vi "ASI_test221128.vi"() -> ()   [LabVIEW 2023]
uses:
  <vilib>/vision/Image Controls.llb/IMAQ Image.ctl
  user.lib/ASICamera2_no_err/ASICamera2_no_err.lvlib
panel:
  in  "live":bool
  out "New Image":T1
  out "Abort":bool
  in  "snap":bool
  in  "abort":bool
  in  "选项卡控件":enum32{"cool", "capture", "setting"}(tab)
  in  "cooler":bool
  in  "set point":i8
  in  "capture num":u16
  in  "imageType":u16(ring)
  in  "bin":u16(ring)
  out "temp and cool chart":cluster{dbl, "plValue out":i32}(graph)
  out "IsCoolerCam":u32
  out "exit":bool
  out "exposure progress":u8(slide) scale=0.0..100.0
  in  "clear ROI":bool
  in  "ROI":bool
  in  "OldCtrlVal[]":cluster{"value":dbl, "auto":bool}[](array[cluster]) {"value" min=-500.0 max=1000.0}
  in  "clusterOldCtrlVal":cluster{"value":dbl, "auto":bool} {"value" min=-500.0 max=1000.0}
  in  "cluster_controlCap":T2
  in  "controlCaps[]":T3(array[cluster])
  out "camera name":string
  in  "newCtrlVal[]":T4(array[cluster])
  in  "cluster":cluster{"name":string, "value":dbl, "auto":bool} {"value" min=-500.0 max=1000.0}
  out "Image":T1(plugin-control)
  out "CameraID":i32
  out "MaxWidth":i32
  out "MaxHeight":i32
  in  "Exit":bool
  in  "iCameraIndex":i32
  out "camera num":i32
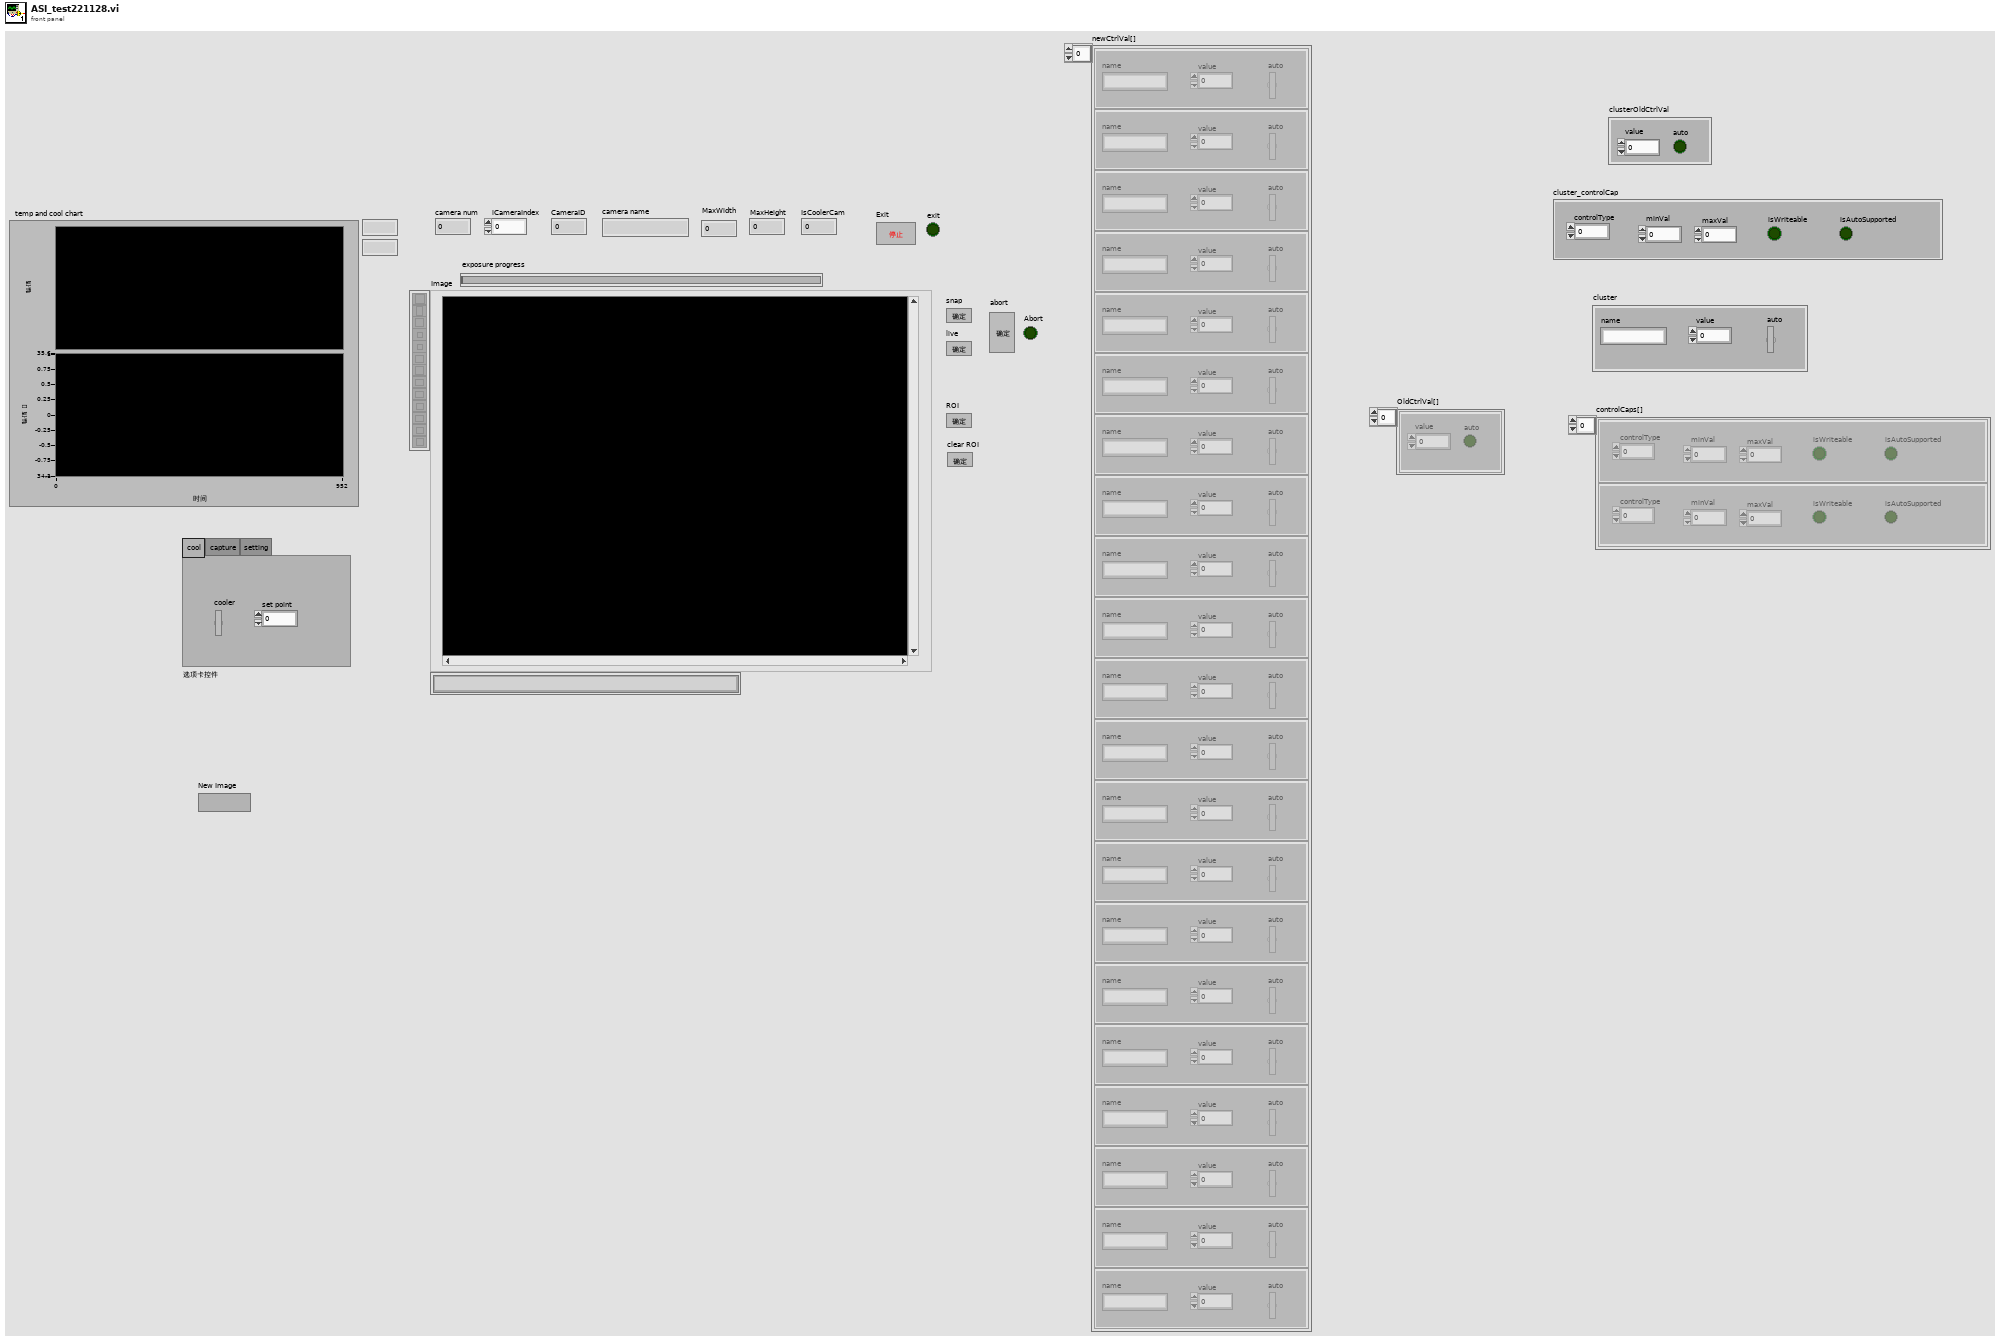
[diagram p1: front panel]
types:
  T1 = typedef "IMAQ Image.ctl" = refnum<image>
  T2 = cluster{"minVal":dbl, "maxVal":dbl, "isWriteable":bool, "isAutoSupported":bool, "controlType":dbl}
  T3 = cluster{"minVal":dbl, "maxVal":dbl, "isWriteable":bool, "isAutoSupported":bool, "controlType":dbl}[]
  T4 = cluster{"name":string, "value":dbl, "auto":bool}[]
  T5 = cluster{"Name[0]":i8, "Name[1]":i8, "Name[2]":i8, "Name[3]":i8, "Name[4]":i8, "Name[5]":i8, "Name[6]":i8, "Name[7]":i8, "Name[8]":i8, "Name[9]":i8, "Name[10]":i8, "Name[11]":i8, "Name[12]":i8, "Name[13]":i8, "Name[14]":i8, "Name[15]":i8, "Name[16]":i8, "Name[17]":i8, "Name[18]":i8, "Name[19]":i8, "Name[20]":i8, "Name[21]":i8, "Name[22]":i8, "Name[23]":i8, "Name[24]":i8, "Name[25]":i8, "Name[26]":i8, "Name[27]":i8, "Name[28]":i8, "Name[29]":i8, "Name[30]":i8, "Name[31]":i8, "Name[32]":i8, "Name[33]":i8, "Name[34]":i8, "Name[35]":i8, "Name[36]":i8, "Name[37]":i8, "Name[38]":i8, "Name[39]":i8, "Name[40]":i8, "Name[41]":i8, "Name[42]":i8, "Name[43]":i8, "Name[44]":i8, "Name[45]":i8, "Name[46]":i8, "Name[47]":i8, "Name[48]":i8, "Name[49]":i8, "Name[50]":i8, "Name[51]":i8, "Name[52]":i8, "Name[53]":i8, "Name[54]":i8, "Name[55]":i8, "Name[56]":i8, "Name[57]":i8, "Name[58]":i8, "Name[59]":i8, "Name[60]":i8, "Name[61]":i8, "Name[62]":i8, "Name[63]":i8, "CameraID":i32, "MaxHeight":i32, "MaxWidth":i32, "IsColorCam":u32, "BayerPattern":u32, "SupportedBins[0]":i32, "SupportedBins[1]":i32, "SupportedBins[2]":i32, "SupportedBins[3]":i32, "SupportedBins[4]":i32, "SupportedBins[5]":i32, "SupportedBins[6]":i32, "SupportedBins[7]":i32, "SupportedBins[8]":i32, "SupportedBins[9]":i32, "SupportedBins[10]":i32, "SupportedBins[11]":i32, "SupportedBins[12]":i32, "SupportedBins[13]":i32, "SupportedBins[14]":i32, "SupportedBins[15]":i32, "SupportedVideoFormat[0]":u32, "SupportedVideoFormat[1]":u32, "SupportedVideoFormat[2]":u32, "SupportedVideoFormat[3]":u32, "SupportedVideoFormat[4]":u32, "SupportedVideoFormat[5]":u32, "SupportedVideoFormat[6]":u32, "SupportedVideoFormat[7]":u32, "@dummy control@":i8, "@dummy control@":i8, "@dummy control@":i8, "@dummy control@":i8, "PixelSize":dbl, "MechanicalShutter":u32, "ST4Port":u32, "IsCoolerCam":u32, "IsUSB3Host":u32, "IsUSB3Camera":u32, "ElecPerADU":sgl, "Unused[0]":i8, "Unused[1]":i8, "Unused[2]":i8, "Unused[3]":i8, "Unused[4]":i8, "Unused[5]":i8, "Unused[6]":i8, "Unused[7]":i8, "Unused[8]":i8, "Unused[9]":i8, "Unused[10]":i8, "Unused[11]":i8, "Unused[12]":i8, "Unused[13]":i8, "Unused[14]":i8, "Unused[15]":i8, "Unused[16]":i8, "Unused[17]":i8, "Unused[18]":i8, "Unused[19]":i8, "Unused[20]":i8, "Unused[21]":i8, "Unused[22]":i8, "Unused[23]":i8}
  T6 = typedef "Image Type" = u32
  T7 = cluster{"Name[0]":i8, "Name[1]":i8, "Name[2]":i8, "Name[3]":i8, "Name[4]":i8, "Name[5]":i8, "Name[6]":i8, "Name[7]":i8, "Name[8]":i8, "Name[9]":i8, "Name[10]":i8, "Name[11]":i8, "Name[12]":i8, "Name[13]":i8, "Name[14]":i8, "Name[15]":i8, "Name[16]":i8, "Name[17]":i8, "Name[18]":i8, "Name[19]":i8, "Name[20]":i8, "Name[21]":i8, "Name[22]":i8, "Name[23]":i8, "Name[24]":i8, "Name[25]":i8, "Name[26]":i8, "Name[27]":i8, "Name[28]":i8, "Name[29]":i8, "Name[30]":i8, "Name[31]":i8, "Name[32]":i8, "Name[33]":i8, "Name[34]":i8, "Name[35]":i8, "Name[36]":i8, "Name[37]":i8, "Name[38]":i8, "Name[39]":i8, "Name[40]":i8, "Name[41]":i8, "Name[42]":i8, "Name[43]":i8, "Name[44]":i8, "Name[45]":i8, "Name[46]":i8, "Name[47]":i8, "Name[48]":i8, "Name[49]":i8, "Name[50]":i8, "Name[51]":i8, "Name[52]":i8, "Name[53]":i8, "Name[54]":i8, "Name[55]":i8, "Name[56]":i8, "Name[57]":i8, "Name[58]":i8, "Name[59]":i8, "Name[60]":i8, "Name[61]":i8, "Name[62]":i8, "Name[63]":i8, "Description[0]":i8, "Description[1]":i8, "Description[2]":i8, "Description[3]":i8, "Description[4]":i8, "Description[5]":i8, "Description[6]":i8, "Description[7]":i8, "Description[8]":i8, "Description[9]":i8, "Description[10]":i8, "Description[11]":i8, "Description[12]":i8, "Description[13]":i8, "Description[14]":i8, "Description[15]":i8, "Description[16]":i8, "Description[17]":i8, "Description[18]":i8, "Description[19]":i8, "Description[20]":i8, "Description[21]":i8, "Description[22]":i8, "Description[23]":i8, "Description[24]":i8, "Description[25]":i8, "Description[26]":i8, "Description[27]":i8, "Description[28]":i8, "Description[29]":i8, "Description[30]":i8, "Description[31]":i8, "Description[32]":i8, "Description[33]":i8, "Description[34]":i8, "Description[35]":i8, "Description[36]":i8, "Description[37]":i8, "Description[38]":i8, "Description[39]":i8, "Description[40]":i8, "Description[41]":i8, "Description[42]":i8, "Description[43]":i8, "Description[44]":i8, "Description[45]":i8, "Description[46]":i8, "Description[47]":i8, "Description[48]":i8, "Description[49]":i8, "Description[50]":i8, "Description[51]":i8, "Description[52]":i8, "Description[53]":i8, "Description[54]":i8, "Description[55]":i8, "Description[56]":i8, "Description[57]":i8, "Description[58]":i8, "Description[59]":i8, "Description[60]":i8, "Description[61]":i8, "Description[62]":i8, "Description[63]":i8, "Description[64]":i8, "Description[65]":i8, "Description[66]":i8, "Description[67]":i8, "Description[68]":i8, "Description[69]":i8, "Description[70]":i8, "Description[71]":i8, "Description[72]":i8, "Description[73]":i8, "Description[74]":i8, "Description[75]":i8, "Description[76]":i8, "Description[77]":i8, "Description[78]":i8, "Description[79]":i8, "Description[80]":i8, "Description[81]":i8, "Description[82]":i8, "Description[83]":i8, "Description[84]":i8, "Description[85]":i8, "Description[86]":i8, "Description[87]":i8, "Description[88]":i8, "Description[89]":i8, "Description[90]":i8, "Description[91]":i8, "Description[92]":i8, "Description[93]":i8, "Description[94]":i8, "Description[95]":i8, "Description[96]":i8, "Description[97]":i8, "Description[98]":i8, "Description[99]":i8, "Description[100]":i8, "Description[101]":i8, "Description[102]":i8, "Description[103]":i8, "Description[104]":i8, "Description[105]":i8, "Description[106]":i8, "Description[107]":i8, "Description[108]":i8, "Description[109]":i8, "Description[110]":i8, "Description[111]":i8, "Description[112]":i8, "Description[113]":i8, "Description[114]":i8, "Description[115]":i8, "Description[116]":i8, "Description[117]":i8, "Description[118]":i8, "Description[119]":i8, "Description[120]":i8, "Description[121]":i8, "Description[122]":i8, "Description[123]":i8, "Description[124]":i8, "Description[125]":i8, "Description[126]":i8, "Description[127]":i8, "MaxValue":i32, "MinValue":i32, "DefaultValue":i32, "IsAutoSupported":u32, "IsWritable":u32, "ControlType":u32, "Unused[0]":i8, "Unused[1]":i8, "Unused[2]":i8, "Unused[3]":i8, "Unused[4]":i8, "Unused[5]":i8, "Unused[6]":i8, "Unused[7]":i8, "Unused[8]":i8, "Unused[9]":i8, "Unused[10]":i8, "Unused[11]":i8, "Unused[12]":i8, "Unused[13]":i8, "Unused[14]":i8, "Unused[15]":i8, "Unused[16]":i8, "Unused[17]":i8, "Unused[18]":i8, "Unused[19]":i8, "Unused[20]":i8, "Unused[21]":i8, "Unused[22]":i8, "Unused[23]":i8, "Unused[24]":i8, "Unused[25]":i8, "Unused[26]":i8, "Unused[27]":i8, "Unused[28]":i8, "Unused[29]":i8, "Unused[30]":i8, "Unused[31]":i8}
  T8 = cluster{"Global Rectangle":i32[], "Contours":cluster{"Contour Type":u32, "ROI Type":u32, "Points":i32[]}[]}
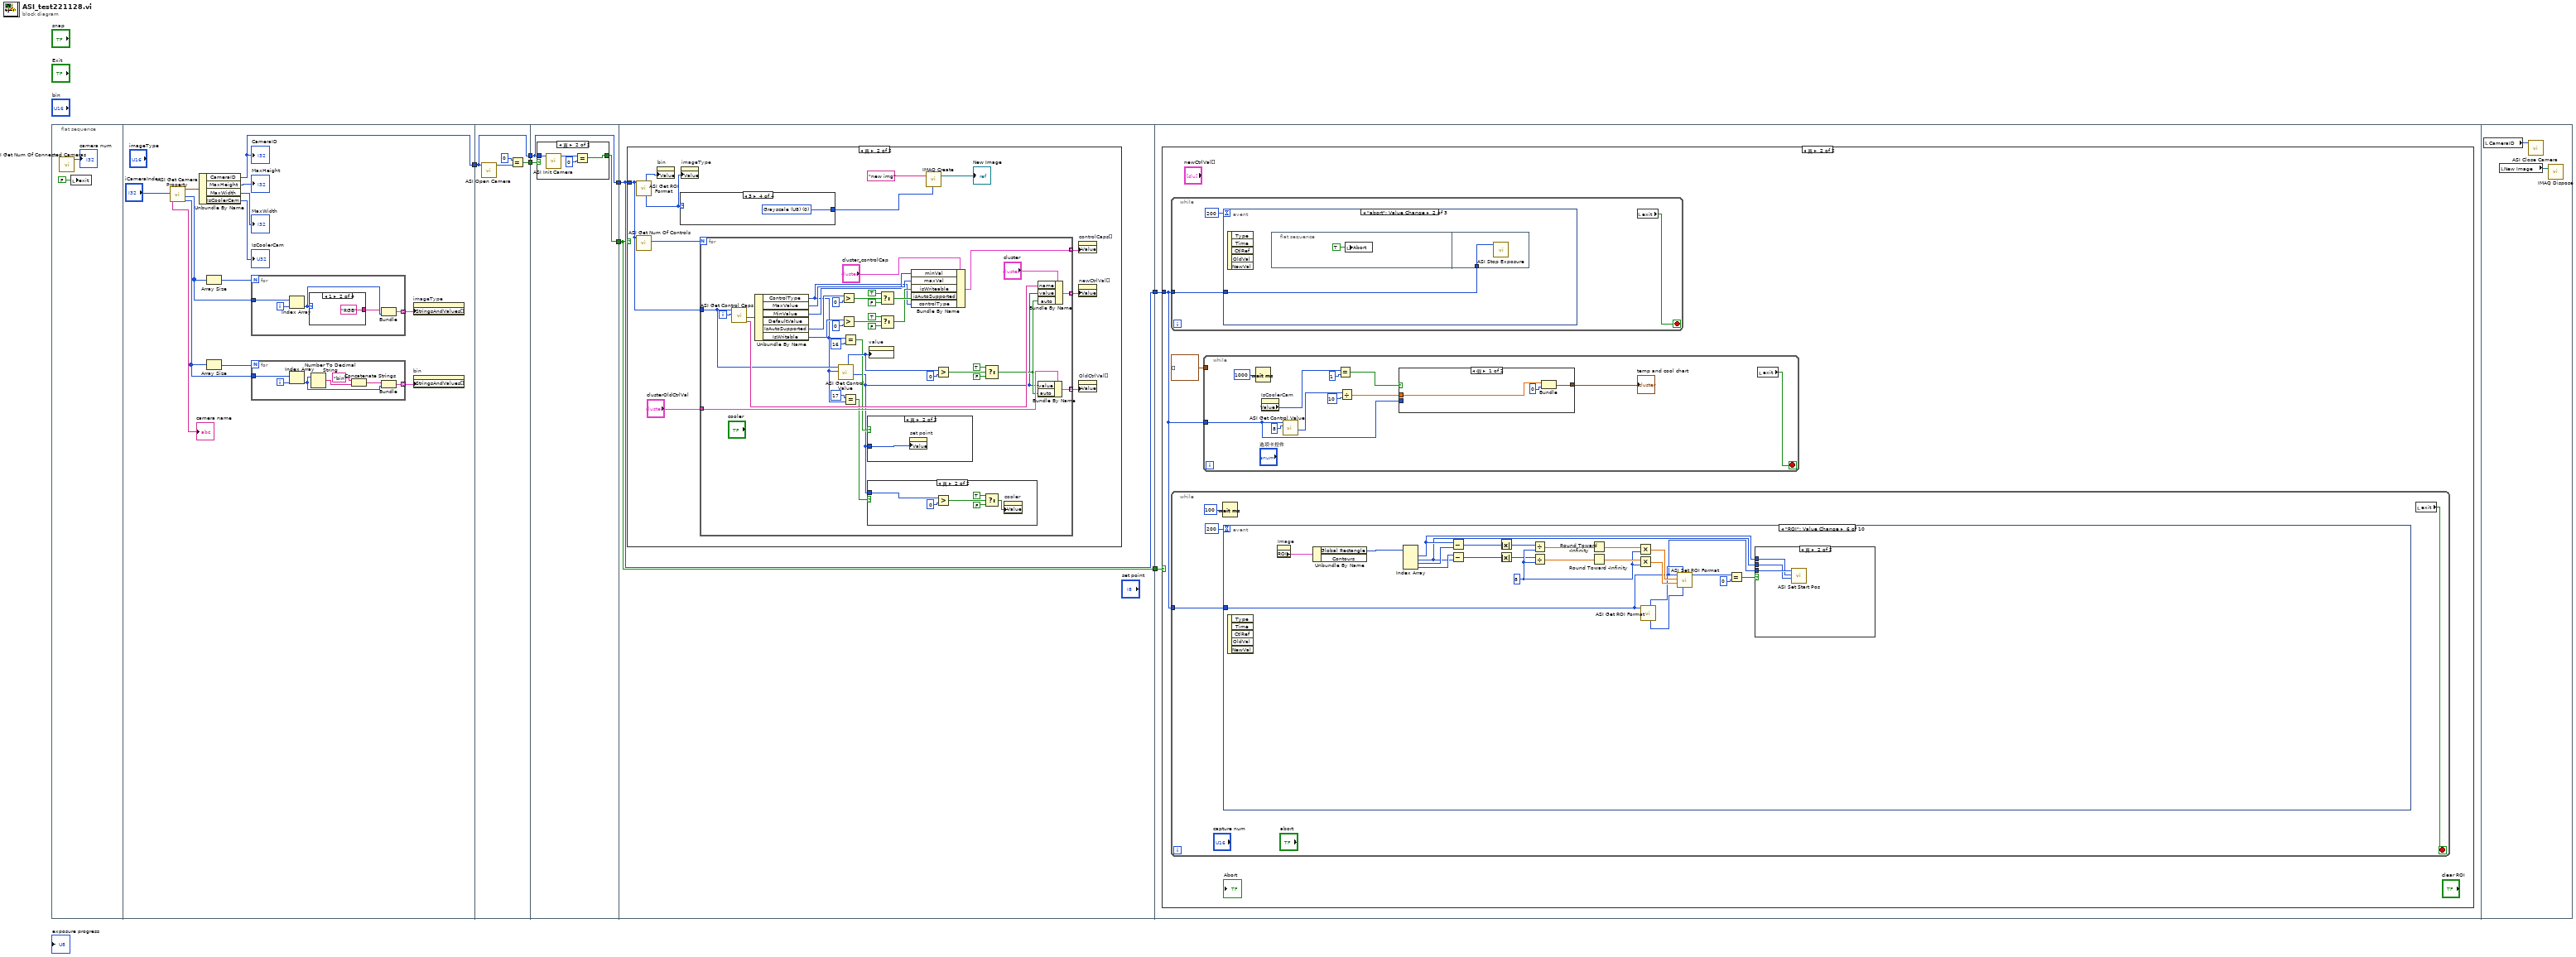
[diagram p0: block diagram]
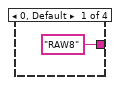
[diagram p2: hidden frame]
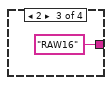
[diagram p3: hidden frame]
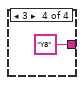
[diagram p4: hidden frame]
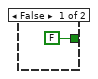
[diagram p5: hidden frame]
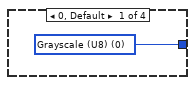
[diagram p7: hidden frame]
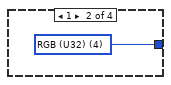
[diagram p8: hidden frame]
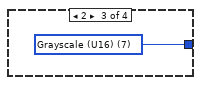
[diagram p9: hidden frame]
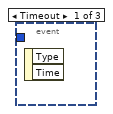
[diagram p13: hidden frame]
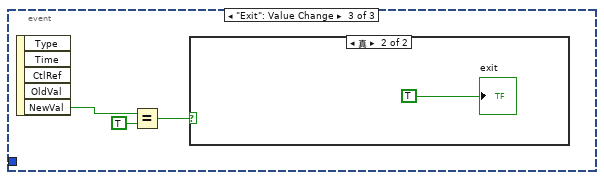
[diagram p14: hidden frame]
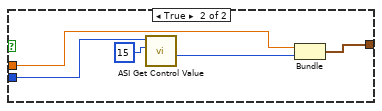
[diagram p16: hidden frame]
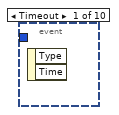
[diagram p17: hidden frame]
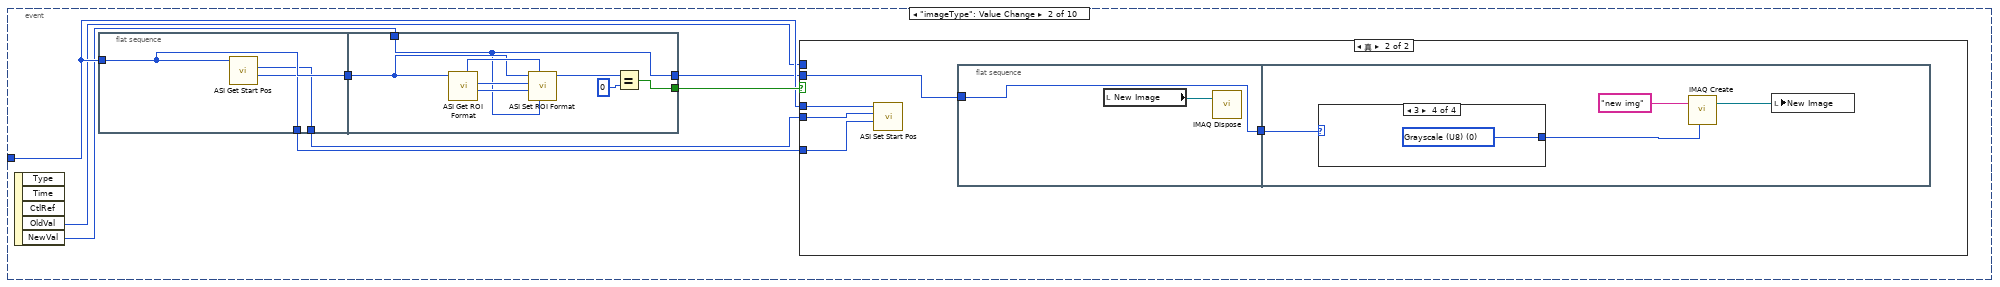
[diagram p18: hidden frame]
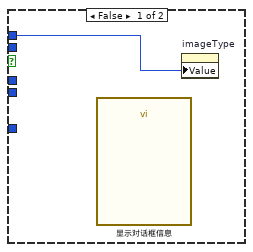
[diagram p19: hidden frame]
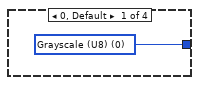
[diagram p20: hidden frame]
diagram:
  n1 = flat-sequence "平铺式顺序结构" {
    tunnel: [w20] -> w7
    tunnel: w7 -> [w42]
    tunnel: [w42] -> w6
    tunnel: [w39] -> w2
    tunnel: w6 -> [w45]
    tunnel: [w45] -> w5
    tunnel: w2 -> [w44]
    tunnel: [w43] -> w1
    tunnel: w5 -> [w52]
    tunnel: [w52] -> w4
    tunnel: [w51] -> w3
    tunnel: w1 -> [w51]
    tunnel: w4 -> [w112]
    tunnel: w3 -> [w111]
    frame #0 {
      n2 = call "ASI Get Num Of Connected Cameras.vi"() -> ("function return"=→"camera num":i32)  [unwired: 10 in, 1 out]
      n3 = local write "exit"(FALSE ("exit")) -> ()
    }
    frame #1 {
      n4 = call "ASI Get Camera Property.vi"("iCameraIndex"="iCameraIndex") -> ("supportedBin"=w15:i8[], "supportedImgType"=w16:i8[], "pASICameraInfo out"=w21:T5, "cameraName"=→"camera name":string)  [unwired: 6 in, 1 out]
      n5 = Unbundle By Name(w21) -> ("CameraID"=w20:i32, "MaxHeight"=→"MaxHeight":i32, "MaxWidth"=→"MaxWidth":i32, "IsCoolerCam"=→"IsCoolerCam":u32)
      "CameraID" <- w20
      n6 = Array Size(array=w16) -> (size(s)=w17:i32)
      n7 = Array Size(array=w15) -> (size(s)=w14:i32)
      n8 = for {
        N: w17 -> [_]
        tunnel: w16 -> [w33]
        tunnel: [w30] -> w11 mode=indexing
        i -> [w34]
        n9 = Index Array(array=w33, index=w34) -> (element=w32:i8)
        n10 = case shown="1" w32 {
          tunnel: ["RAW8" "RGB" "RAW16" "Y8"] -> w31
          frame 0, Default {
          }
          frame 1 {
          }
          frame 2 {
          }
          frame 3 {
          }
        }
        n11 = Bundle(w31, "SupportedVideoFormat[6]"=w32) -> (w30:cluster{string, "SupportedVideoFormat[6]":i8})  [unwired: 1 in]
      }
      n12 = for {
        N: w14 -> [_]
        tunnel: w15 -> [w28]
        tunnel: [w23] -> w13 mode=indexing
        i -> [w29]
        n13 = Index Array(array=w28, index=w29) -> (element=w27:i8)
        n14 = Number To Decimal String(number=w27) -> (decimal integer string=w25:string)  [unwired: 1 in]
        n15 = Concatenate Strings("bin" ("字符串"), w25) -> (w24:string)
        n16 = Bundle(w24, "元素"=w27) -> (w23:cluster{string, "元素":i8})  [unwired: 1 in]
      }
      n17 = property on="imageType" class="Ring (strict)"("StringsAndValues[]"=w11) -> ()  [unwired: 2 in, 2 out]
      n18 = property on="bin" class="Ring (strict)"("StringsAndValues[]"=w13) -> ()  [unwired: 2 in, 2 out]
    }
    frame #2 {
      n19 = call "ASI Open Camera.vi"("iCameraID"=w42) -> ("function return"=w41:i32)  [unwired: 10 in]
      n20 = Equal?(x=0, y=w41) -> (x = y?=w39:bool)
    }
    frame #3 {
      n21 = case shown="真" w44 {
        tunnel: w45 -> [_ w50]
        tunnel: [FALSE w47] -> w43
        frame False {
        }
        frame True {
          n22 = call "ASI Init Camera.vi"("iCameraID"=w50) -> ("function return"=w48:i32)  [unwired: 10 in]
          n23 = Equal?(x=w48, y=0 ("x")) -> (x = y?=w47:bool)
        }
      }
    }
    frame #4 {
      n24 = case shown="真" w51 {
        tunnel: w52 -> [_ w62]
        frame False {
        }
        frame True {
          n25 = call "ASI Get ROI Format.vi"("iCameraID"=w62) -> ("pImg_type out"=w54:i32, "piBin out"=w61:i32)  [unwired: 6 in, 3 out]
          n26 = call "ASI Get Num Of Controls.vi"("iCameraID"=w62) -> ("piNumberOfControls out"=w63:i32)  [unwired: 9 in, 1 out]
          n27 = property on="bin" class="Ring (strict)"("Value"=w61) -> ()  [unwired: 2 in, 2 out]
          n28 = case shown="3" w54 {
            tunnel: [w64 w65 w66 w67] -> w56
            frame 0, Default {
              w64 = T6 0 items=["Grayscale (U8)", "Grayscale (I16)", "Grayscale (SGL)", "Complex (CSG)", "RGB (U32)", "HSL (U32)", "RGB (U64)", "Grayscale (U16)"] ("Image Type")
            }
            frame 1 {
              w65 = T6 4 items=["Grayscale (U8)", "Grayscale (I16)", "Grayscale (SGL)", "Complex (CSG)", "RGB (U32)", "HSL (U32)", "RGB (U64)", "Grayscale (U16)"] ("Image Type")
            }
            frame 2 {
              w66 = T6 7 items=["Grayscale (U8)", "Grayscale (I16)", "Grayscale (SGL)", "Complex (CSG)", "RGB (U32)", "HSL (U32)", "RGB (U64)", "Grayscale (U16)"] ("Image Type")
            }
            frame 3 {
              w67 = T6 0 items=["Grayscale (U8)", "Grayscale (I16)", "Grayscale (SGL)", "Complex (CSG)", "RGB (U32)", "HSL (U32)", "RGB (U64)", "Grayscale (U16)"] ("Image Type")
            }
          }
          n29 = property on="imageType" class="Ring (strict)"("Value"=w54) -> ()  [unwired: 2 in, 2 out]
          n30 = for {
            N: w63 -> [_]
            tunnel: w62 -> [w100]
            tunnel: [w75] -> w60 mode=indexing
            tunnel: [w76] -> w59 mode=indexing
            tunnel: "clusterOldCtrlVal" -> [w79]
            tunnel: [w74] -> w57 mode=indexing
            i -> [w78]
            n31 = call "ASI Get Control Caps.vi"("iControlIndex"=w78, "iCameraID"=w100) -> ("name"=w101:string, "pControlCaps out"=w103:T7)  [unwired: 7 in, 1 out]
            n32 = Unbundle By Name(w103) -> ("ControlType"=w71:u32, "MaxValue"=w93:i32, "MinValue"=w92:i32, "IsAutoSupported"=w89:u32, "IsWritable"=w82:u32)  [unwired: 1 out]
            n33 = call "ASI Get Control Value.vi"("ControlType"=w71, "iCameraID"=w100) -> ("plValue out"=w68:i32, "pbAuto out"=w95:i32)  [unwired: 7 in, 1 out]
            n34 = Greater?(x=w89, y=u32 0) -> (0:w87:bool)
            n35 = Greater?(x=w82, y=u32 0) -> (0:w81:bool)
            n36 = Equal?(x=w71, y=u32 16) -> (x = y?=w69:bool)
            n37 = Equal?(x=u32 17, y=w71) -> (x = y?=w72:bool)
            n38 = case shown="真" w69 {
              tunnel: w68 -> [_ w104]
              frame False {
              }
              frame True {
                n39 = property on="set point" class="DigNum (strict)"("Value"=w104) -> ()  [unwired: 2 in, 2 out]
              }
            }
            n40 = case shown="真" w72 {
              tunnel: w68 -> [_ w106]
              frame False {
              }
              frame True {
                n41 = Greater?(x=w106, y=0) -> (0:w108:bool)
                n42 = Select(t=TRUE, s=w108, f=FALSE) -> (s? t:f=w105:bool)
                n43 = property on="cooler" class="Bool (strict)"("Value"=w105) -> ()  [unwired: 2 in, 2 out]
              }
            }
            n44 = property on="value" class="DigNum (strict)"("DisabledEnum"=w95) -> ()  [unwired: 2 in, 2 out]
            n45 = Select(t=TRUE, s=w87, f=FALSE) -> (s? t:f=w86:bool)
            n46 = Select(t=TRUE, s=w81, f=FALSE) -> (s? t:f=w80:bool)
            n47 = Bundle By Name(cluster="cluster_controlCap", "minVal"=w92, "maxVal"=w93, "isWriteable"=w80, "isAutoSupported"=w86, "controlType"=w71) -> (w76:T2)
            n48 = Greater?(x=w95, y=0) -> (0:w99:bool)
            n49 = Select(t=TRUE, s=w99, f=FALSE) -> (s? t:f=w77:bool)
            n50 = Bundle By Name(cluster="cluster", "name"=w101, "value"=w68, "auto"=w77) -> (w75:cluster{"name":string, "value":dbl, "auto":bool})
            n51 = Bundle By Name(cluster=w79, "value"=w68, "auto"=w77) -> (w74:cluster{"value":dbl, "auto":bool})
          }
          n52 = call "IMAQ Create"("Image Name"="new img", "Image Type"=w56) -> ("New Image"=→"New Image":T1)  [unwired: 3 in, 1 out]
          n53 = property on="controlCaps[]" class="Arr (strict)"("Value"=w59) -> ()  [unwired: 2 in, 2 out]
          n54 = property on="newCtrlVal[]" class="Arr (strict)"("Value"=w60) -> ()  [unwired: 2 in, 2 out]
          n55 = property on="OldCtrlVal[]" class="Arr (strict)"("Value"=w57) -> ()  [unwired: 2 in, 2 out]
        }
      }
    }
    frame #5 {
      n56 = case shown="真" w111 {
        tunnel: w112 -> [_ w114]
        frame False {
        }
        frame True {
          n57 = while {
            tunnel: w114 -> [w117]
            stop <- w115 stop-if-true
            n58 = event shown="[1] \"abort\": Value Change" {
              selector: _ -> [_ _ _]
              dyn-events: _ -> [_ _ _]
              timeout: 200 -> [_ _ _]
              tunnel: w117 -> [_ w118 _]
              event Timeout {
                n59 = event-data() -> ()  [unwired: 1 in, 2 out]
              }
              event "abort": Value Change {
                n60 = event-data() -> ()  [unwired: 1 in, 5 out]
                n61 = flat-sequence {
                  tunnel: w118 -> [w120]
                  frame #0 {
                    n62 = local write "Abort"(TRUE ("exit")) -> ()
                  }
                  frame #1 {
                    n63 = call "ASI Stop Exposure.vi"("iCameraID"=w120) -> ()  [unwired: 10 in, 1 out]
                  }
                }
              }
              event "Exit": Value Change {
                n64 = event-data() -> ("NewVal"=w123:bool)  [unwired: 1 in, 4 out]
                n65 = Equal?(x=w123, y=TRUE) -> (x = y?=w121:bool)
                n66 = case shown="真" w121 {
                  frame False {
                  }
                  frame True {
                    "exit" <- TRUE ("exit")
                  }
                }
              }
            }
            n67 = local read "exit"() -> (w115:bool)
          }
          n68 = while {
            tunnel: w114 -> [w146]
            stop <- w144 stop-if-true
            n69 = Wait (ms)(milliseconds to wait=u32 100 ("等待时间（毫秒）")) -> ()  [unwired: 1 out]
            n70 = event shown="[5] \"ROI\": Value Change" {
              selector: _ -> [_ _ _ _ _ _ _ _ _ _]
              dyn-events: _ -> [_ _ _ _ _ _ _ _ _ _]
              timeout: 200 -> [_ _ _ _ _ _ _ _ _ _]
              tunnel: w146 -> [_ w154 w186 w218 w272 w314 w347 w358 w367 w373]
              event Timeout {
                n71 = event-data() -> ()  [unwired: 1 in, 2 out]
              }
              event "imageType": Value Change {
                n72 = event-data() -> ("OldVal"=w149:u16, "NewVal"=w150:u16)  [unwired: 1 in, 3 out]
                n73 = flat-sequence {
                  tunnel: w154 -> [w158]
                  tunnel: [w158] -> w153
                  tunnel: [w157] -> w152
                  tunnel: [w156] -> w151
                  tunnel: [w162] -> w155
                  tunnel: w153 -> [w160]
                  tunnel: w150 -> [w159]
                  tunnel: [w159] -> w148
                  frame #0 {
                    n74 = call "ASI Get Start Pos.vi"("iCameraID"=w158) -> ("piStartY out"=w156:i32, "piStartX out"=w157:i32)  [unwired: 8 in, 1 out]
                  }
                  frame #1 {
                    n75 = call "ASI Get ROI Format.vi"("iCameraID"=w160) -> ("piHeight out"=w165:i32, "piWidth out"=w166:i32, "piBin out"=w164:i32)  [unwired: 6 in, 2 out]
                    n76 = call "ASI Set ROI Format.vi"("Img_type"=w159, "iBin"=w164, "iHeight"=w165, "iWidth"=w166, "iCameraID"=w160) -> ("function return"=w161:i32)  [unwired: 6 in]
                    n77 = Equal?(x=w161, y=u8 0) -> (x = y?=w162:bool)
                  }
                }
                n78 = case shown="真" w155 {
                  tunnel: w154 -> [_ w172]
                  tunnel: w152 -> [_ w171]
                  tunnel: w151 -> [_ w170]
                  tunnel: w149 -> [w167 _]
                  tunnel: w148 -> [_ w169]
                  frame False {
                    n79 = call "显示对话框信息"() -> ()  [unwired: 10 in, 2 out]
                    n80 = property on="imageType" class="Ring (strict)"("Value"=w167) -> ()  [unwired: 2 in, 2 out]
                  }
                  frame True {
                    n81 = call "ASI Set Start Pos.vi"("iStartY"=w170, "iStartX"=w171, "iCameraID"=w172) -> ()  [unwired: 8 in, 1 out]
                    n82 = flat-sequence {
                      tunnel: w169 -> [w174]
                      tunnel: [w174] -> w168
                      tunnel: w168 -> [w176]
                      frame #0 {
                        n83 = local read "New Image"() -> (w173:T1)
                        n84 = call "IMAQ Dispose"("Image"=w173) -> ()  [unwired: 5 in, 1 out]
                      }
                      frame #1 {
                        n85 = case shown="3" w176 {
                          tunnel: [w179 w180 w181 w182] -> w178
                          frame 0, Default {
                            w179 = T6 0 items=["Grayscale (U8)", "Grayscale (I16)", "Grayscale (SGL)", "Complex (CSG)", "RGB (U32)", "HSL (U32)", "RGB (U64)", "Grayscale (U16)"] ("Image Type")
                          }
                          frame 1 {
                            w180 = T6 4 items=["Grayscale (U8)", "Grayscale (I16)", "Grayscale (SGL)", "Complex (CSG)", "RGB (U32)", "HSL (U32)", "RGB (U64)", "Grayscale (U16)"] ("Image Type")
                          }
                          frame 2 {
                            w181 = T6 7 items=["Grayscale (U8)", "Grayscale (I16)", "Grayscale (SGL)", "Complex (CSG)", "RGB (U32)", "HSL (U32)", "RGB (U64)", "Grayscale (U16)"] ("Image Type")
                          }
                          frame 3 {
                            w182 = T6 0 items=["Grayscale (U8)", "Grayscale (I16)", "Grayscale (SGL)", "Complex (CSG)", "RGB (U32)", "HSL (U32)", "RGB (U64)", "Grayscale (U16)"] ("Image Type")
                          }
                        }
                        n86 = call "IMAQ Create"("Image Name"="new img", "Image Type"=w178) -> ("New Image"=w175:T1)  [unwired: 3 in, 1 out]
                        n87 = local write "New Image"(w175) -> ()
                      }
                    }
                  }
                }
              }
              event "bin": Value Change {
                w190 = u16 8 ("y")
                n88 = event-data() -> ("OldVal"=w183:u16, "NewVal"=w184:u16)  [unwired: 1 in, 3 out]
                n89 = call "ASI Get ROI Format.vi"("iCameraID"=w186) -> ("piHeight out"=w201:i32, "piWidth out"=w203:i32, "pImg_type out"=w199:i32, "piBin out"=w185:i32)  [unwired: 6 in, 1 out]
                n90 = Multiply(x=w203, y=w185) -> (x*y=w202:i32)
                n91 = Multiply(x=w201, y=w185) -> (x*y=w200:i32)
                n92 = Divide(x=w202, y=w184) -> (x/y=w198:dbl)
                n93 = Divide(x=w200, y=w184) -> (x/y=w193:dbl)
                n94 = Divide(x=w198, y=w190) -> (x/y=w197:dbl)
                n95 = Divide(x=w193, y=w190) -> (x/y=w195:dbl)
                n96 = Round Toward -Infinity(1:w197) -> (0:w196:dbl)
                n97 = Round Toward -Infinity(1:w195) -> (0:w194:dbl)
                n98 = Multiply(x=w196, y=w190) -> (x*y=w191:dbl)
                n99 = Multiply(x=w194, y=w190) -> (x*y=w192:dbl)
                n100 = call "ASI Set ROI Format.vi"("Img_type"=w199, "iBin"=w184, "iHeight"=w192, "iWidth"=w191, "iCameraID"=w186) -> ("function return"=w187:i32)  [unwired: 6 in]
                n101 = Equal?(x=w187, y=u8 0) -> (x = y?=w188:bool)
                n102 = case shown="假" w188 {
                  tunnel: w186 -> [w213 _]
                  tunnel: w184 -> [w210 _]
                  tunnel: w185 -> [w209 _]
                  tunnel: w183 -> [w204 _]
                  frame False {
                    n103 = property on="bin" class="Ring (strict)"("Value"=w204) -> ()  [unwired: 2 in, 2 out]
                    n104 = call "显示对话框信息2"() -> ()  [unwired: 10 in, 2 out]
                    n105 = call "ASI Get Start Pos.vi"("iCameraID"=w213) -> ("piStartY out"=w207:i32, "piStartX out"=w208:i32)  [unwired: 8 in, 1 out]
                    n106 = Multiply(x=w208, y=w209) -> (x*y=w212:i32)
                    n107 = Multiply(x=w207, y=w209) -> (x*y=w211:i32)
                    n108 = Divide(x=w212, y=w210) -> (x/y=w206:dbl)
                    n109 = Divide(x=w211, y=w210) -> (x/y=w205:dbl)
                    n110 = call "ASI Set Start Pos.vi"("iStartY"=w205, "iStartX"=w206, "iCameraID"=w213) -> ()  [unwired: 8 in, 1 out]
                  }
                  frame True {
                  }
                }
              }
              event "snap": Value Change {
                n111 = event-data() -> ()  [unwired: 1 in, 5 out]
                n112 = call "ASI Get ROI Format.vi"("iCameraID"=w218) -> ("piHeight out"=w215:i32, "piWidth out"=w216:i32, "pImg_type out"=w214:i32)  [unwired: 6 in, 2 out]
                n113 = while {
                  tunnel: w218 -> [w231]
                  tunnel: w216 -> [w224]
                  tunnel: w215 -> [w223]
                  tunnel: w214 -> [w222]
                  i -> [w229]
                  stop <- w226 stop-if-true
                  n114 = call "ASI Start Exposure.vi"("iCameraID"=w231) -> ()  [unwired: 10 in, 1 out]
                  n115 = property on="capture num" class="DigNum (strict)"() -> ("Value"=w230:u16)  [unwired: 2 in, 2 out]
                  n116 = flat-sequence {
                    tunnel: w231 -> [w235]
                    tunnel: [w234] -> w221
                    frame #0 {
                      n117 = call "ASI Get Control Value.vi"("ControlType"=1, "iCameraID"=w235) -> ("plValue out"=w234:i32)  [unwired: 7 in, 2 out]
                    }
                  }
                  n118 = Increment(x=w229) -> (x+1=w228:i32)
                  n119 = Greater Or Equal?(x=w228, y=w230) -> (x >= y?=w227:bool)
                  n120 = while {
                    tunnel: w231 -> [w249]
                    tunnel: [w246] -> w220
                    tunnel: w221 -> [w241]
                    i -> [w245]
                    stop <- w247 stop-if-true
                    w236 = u8 98 ("y")
                    w244 = u32 50 ("等待时间（毫秒）")
                    n121 = call "ASI Get Exp Status.vi"("iCameraID"=w249) -> ("pExpStatus out"=w246:u32)  [unwired: 9 in, 1 out]
                    n122 = Wait (ms)(milliseconds to wait=w244) -> ()  [unwired: 1 out]
                    n123 = Not Equal?(x=u32 1, y=w246) -> (x != y?=w247:bool)
                    n124 = Multiply(x=w244, y=w245) -> (x*y=w242:u32)
                    n125 = Multiply(x=w242, y=u32 100000) -> (x*y=w240:u32)
                    n126 = Divide(x=w240, y=w241) -> (x/y=w238:dbl)
                    n127 = Greater Or Equal?(x=w238, y=w236) -> (x >= y?=w239:bool)
                    n128 = Select(t=w236, s=w239, f=w238) -> (s? t:f=w237:dbl)
                    n129 = property on="exposure progress" class="Slide (strict)"("Value"=w237) -> ()  [unwired: 2 in, 2 out]
                  }
                  n130 = local read "Abort"() -> (w225:bool)
                  n131 = Or(x=w227, y=w225) -> (x .or. y?=w226:bool)
                  n132 = Equal?(x=u32 2, y=w220) -> (x = y?=w232:bool)
                  n133 = case shown="真" w232 {
                    tunnel: w231 -> [_ w259]
                    tunnel: w224 -> [_ w255]
                    tunnel: w223 -> [_ w254]
                    tunnel: w222 -> [_ w253]
                    tunnel: w222 -> [_ w252]
                    frame False {
                    }
                    frame True {
                      n134 = flat-sequence {
                        frame #0 {
                          n135 = property on="exposure progress" class="Slide (strict)"("Value"=u8 100 ("exposure progress")) -> ()  [unwired: 2 in, 2 out]
                        }
                        frame #1 {
                          n136 = property on="exposure progress" class="Slide (strict)"("Value"=u8 0 ("exposure progress")) -> ()  [unwired: 2 in, 2 out]
                        }
                      }
                      n137 = Multiply(x=w255, y=w254) -> (x*y=w257:i32)
                      n138 = case shown="1" w252 {
                        tunnel: w257 -> [w262 w265 w268 w269]
                        tunnel: [w262 w263 w266 w269] -> w258
                        frame 0, Default {
                        }
                        frame 1 {
                          n139 = Multiply(x=w265, y=3) -> (x*y=w263:i32)
                        }
                        frame 2 {
                          n140 = Multiply(x=w268, y=2) -> (x*y=w266:i32)
                        }
                        frame 3 {
                        }
                      }
                      n141 = local read "New Image"() -> (w250:T1)
                      n142 = call "ASI Get Data After Exp.vi"("lBuffSize"=w258, "iCameraID"=w259) -> ("pBuffer out"=w256:u8[])  [unwired: 8 in, 1 out]
                      n143 = call "ASI_bufferToImage.vi"("iWidth"=w255, "iHeight"=w254, "New Image"=w250, "imageType"=w253, "pBuffer in"=w256) -> ("Image"=→"Image":T1)  [unwired: 10 in]
                    }
                  }
                }
                n144 = property on="Abort" class="Bool (strict)"("Value"=FALSE ("abort")) -> ()  [unwired: 2 in, 2 out]
              }
              event "live": Value Change {
                n145 = event-data() -> ()  [unwired: 1 in, 5 out]
                n146 = flat-sequence {
                  tunnel: w272 -> [w280]
                  tunnel: [w280] -> w270
                  frame #0 {
                    n147 = call "ASI Start Video Capture.vi"("iCameraID"=w280) -> ()  [unwired: 10 in, 1 out]
                  }
                }
                n148 = property on="Abort" class="Bool (strict)"("Value"=FALSE ("abort")) -> ()  [unwired: 2 in, 2 out]
                n149 = call "ASI Get ROI Format.vi"("iCameraID"=w270) -> ("piHeight out"=w276:i32, "piWidth out"=w277:i32, "pImg_type out"=w275:i32)  [unwired: 6 in, 2 out]
                n150 = Multiply(x=w277, y=w276) -> (x*y=w279:i32)
                n151 = case shown="1" w275 {
                  tunnel: w279 -> [w282 w285 w288 w289]
                  tunnel: [w282 w283 w286 w289] -> w278
                  frame 0, Default {
                  }
                  frame 1 {
                    n152 = Multiply(x=w285, y=3) -> (x*y=w283:i32)
                  }
                  frame 2 {
                    n153 = Multiply(x=w288, y=2) -> (x*y=w286:i32)
                  }
                  frame 3 {
                  }
                }
                n154 = local read "New Image"() -> (w274:T1)
                n155 = while {
                  tunnel: w270 -> [w300]
                  tunnel: w278 -> [w299]
                  tunnel: w277 -> [w297]
                  tunnel: w276 -> [w296]
                  tunnel: w275 -> [w294]
                  tunnel: w274 -> [w293]
                  tunnel: [w292] -> w271
                  stop <- w301 stop-if-true
                  n156 = call "ASI Get Video Data.vi"("iWaitms"=10, "lBuffSize"=w299, "iCameraID"=w300) -> ("pBuffer out"=w295:u8[], "function return"=w292:i32)  [unwired: 7 in]
                  n157 = Equal?(x=w292, y=0) -> (x = y?=w290:bool)
                  n158 = case shown="真" w290 {
                    tunnel: w297 -> [_ w307]
                    tunnel: w296 -> [_ w306]
                    tunnel: w295 -> [_ w305]
                    tunnel: w294 -> [_ w304]
                    tunnel: w293 -> [_ w302]
                    frame False {
                    }
                    frame True {
                      n159 = call "ASI_bufferToImage.vi"("iWidth"=w307, "iHeight"=w306, "New Image"=w302, "imageType"=w304, "pBuffer in"=w305) -> ("Image"=w303:T1)  [unwired: 10 in]
                      n160 = local write "Image"(w303) -> ()
                    }
                  }
                  n161 = local read "Abort"() -> (w301:bool)
                }
                n162 = flat-sequence {
                  tunnel: w270 -> [w281]
                  tunnel: w271 -> [_]
                  frame #0 {
                    n163 = call "ASI Stop Video Capture.vi"("iCameraID"=w281) -> ()  [unwired: 10 in, 1 out]
                  }
                }
              }
              event "ROI": Value Change {
                w321 = u16 8 ("y")
                n164 = event-data() -> ()  [unwired: 1 in, 5 out]
                n165 = property on="Image" class="ImageControl"() -> ("ROI"=w330:T8)  [unwired: 2 in, 2 out]
                n166 = Unbundle By Name(w330) -> ("Global Rectangle"=w327:i32[])  [unwired: 1 out]
                n167 = Index Array(array=w327) -> (element #1=w313:i32, element #2=w312:i32, element #3=w326:i32, element #4=w319:i32)  [unwired: 4 in]
                n168 = Subtract(x=w313, y=w326) -> (x-y=w311:i32)
                n169 = Subtract(x=w319, y=w312) -> (x-y=w309:i32)
                n170 = Absolute Value(x=w311) -> (abs(x)=w310:i32)
                n171 = Absolute Value(x=w309) -> (abs(x)=w308:i32)
                n172 = Divide(x=w310, y=w321) -> (x/y=w325:dbl)
                n173 = Divide(x=w308, y=w321) -> (x/y=w323:dbl)
                n174 = Round Toward -Infinity(1:w325) -> (0:w324:dbl)
                n175 = Round Toward -Infinity(1:w323) -> (0:w322:dbl)
                n176 = Multiply(x=w324, y=w321) -> (x*y=w320:dbl)
                n177 = Multiply(x=w322, y=w321) -> (x*y=w318:dbl)
                n178 = call "ASI Get ROI Format.vi"("iCameraID"=w314) -> ("pImg_type out"=w317:i32, "piBin out"=w316:i32)  [unwired: 6 in, 3 out]
                n179 = call "ASI Set ROI Format.vi"("Img_type"=w317, "iBin"=w316, "iHeight"=w318, "iWidth"=w320, "iCameraID"=w314) -> ("function return"=w315:i32)  [unwired: 6 in]
                n180 = Equal?(x=w315, y=u8 0) -> (x = y?=w328:bool)
                n181 = case shown="真" w328 {
                  tunnel: w314 -> [_ w333]
                  tunnel: w313 -> [_ w332]
                  tunnel: w312 -> [_ w331]
                  frame False {
                    n182 = call "显示对话框信息3"() -> ()  [unwired: 10 in, 2 out]
                  }
                  frame True {
                    n183 = call "ASI Set Start Pos.vi"("iStartY"=w331, "iStartX"=w332, "iCameraID"=w333) -> ()  [unwired: 8 in, 1 out]
                  }
                }
              }
              event "clear ROI": Value Change {
                w337 = u8 8 ("y")
                n184 = event-data() -> ()  [unwired: 1 in, 5 out]
                n185 = local read "MaxHeight"() -> (w338:i32)
                n186 = local read "MaxWidth"() -> (w346:i32)
                n187 = property on="bin" class="Ring (strict)"() -> ("Value"=w334:u16)  [unwired: 2 in, 2 out]
                n188 = Divide(x=w338, y=w334) -> (x/y=w341:dbl)
                n189 = Divide(x=w346, y=w334) -> (x/y=w345:dbl)
                n190 = Divide(x=w341, y=w337) -> (x/y=w340:dbl)
                n191 = Divide(x=w345, y=w337) -> (x/y=w344:dbl)
                n192 = Round Toward -Infinity(1:w340) -> (0:w339:dbl)
                n193 = Round Toward -Infinity(1:w344) -> (0:w343:dbl)
                n194 = property on="imageType" class="Ring (strict)"() -> ("Value"=w335:u16)  [unwired: 2 in, 2 out]
                n195 = Multiply(x=w339, y=w337) -> (x*y=w336:dbl)
                n196 = Multiply(x=w343, y=w337) -> (x*y=w342:dbl)
                n197 = call "ASI Set ROI Format.vi"("Img_type"=w335, "iBin"=w334, "iHeight"=w336, "iWidth"=w342, "iCameraID"=w347) -> ()  [unwired: 6 in, 1 out]
              }
              event "cooler": Value Change {
                n198 = event-data() -> ("OldVal"=w348:bool, "NewVal"=w356:bool)  [unwired: 1 in, 3 out]
                n199 = Select(t=u8 1, s=w356, f=u8 0) -> (s? t:f=w353:u8)
                n200 = call "ASI Set Control Value.vi"("bAuto"=0, "lValue"=w353, "ControlType"=17, "iCameraID"=w358) -> ("function return"=w351:i32)  [unwired: 7 in]
                n201 = Not Equal?(x=w351, y=0) -> (x != y?=w349:bool)
                n202 = case shown="真" w349 {
                  tunnel: w348 -> [_ w359]
                  frame False {
                  }
                  frame True {
                    n203 = property on="cooler" class="Bool (strict)"("Value"=w359) -> ()  [unwired: 2 in, 2 out]
                  }
                }
              }
              event "set point": Value Change {
                n204 = event-data() -> ("OldVal"=w360:i8, "NewVal"=w365:i8)  [unwired: 1 in, 3 out]
                n205 = call "ASI Set Control Value.vi"("bAuto"=0, "lValue"=w365, "ControlType"=16, "iCameraID"=w367) -> ("function return"=w363:i32)  [unwired: 7 in]
                n206 = Not Equal?(x=w363, y=0) -> (x != y?=w361:bool)
                n207 = case shown="真" w361 {
                  tunnel: w360 -> [_ w368]
                  frame False {
                  }
                  frame True {
                    n208 = property on="set point" class="DigNum (strict)"("Value"=w368) -> ()  [unwired: 2 in, 2 out]
                  }
                }
              }
              event "newCtrlVal[]": Value Change {
                n209 = event-data() -> ("NewVal"=w369:T4)  [unwired: 1 in, 4 out]
                n210 = Array Size(array=w369) -> (size(s)=w375:i32)
                n211 = for {
                  N: w375 -> [_]
                  tunnel: w369 -> [w378]
                  tunnel: "OldCtrlVal[]" -> [w396]
                  tunnel: "controlCaps[]" -> [w393]
                  tunnel: w373 -> [w388]
                  tunnel: w373 -> [w383]
                  tunnel: [w377] -> w371 mode=indexing
                  tunnel: [w376] -> w370 mode=indexing
                  i -> [w384]
                  n212 = Index Array(array=w396, index=w384) -> (element=w394:cluster{"value":dbl, "auto":bool})
                  n213 = Index Array(array=w378, index=w384) -> (element=w395:cluster{"name":string, "value":dbl, "auto":bool})
                  n214 = Unbundle By Name(w394) -> ("value"=w387:dbl, "auto"=w380:bool)
                  n215 = Unbundle By Name(w395) -> ("name"=w379:string, "value"=w386:dbl, "auto"=w381:bool)
                  n216 = Index Array(array=w393, index=w384) -> (element=w392:T2)
                  n217 = Unbundle By Name(w392) -> ("isWriteable"=w385:bool, "isAutoSupported"=w390:bool, "controlType"=w382:dbl)
                  n218 = Not Equal?(x=w381, y=w380) -> (x != y?=w391:bool)
                  n219 = And(x=w391, y=w390) -> (x .and. y?=w389:bool)
                  n220 = flat-sequence {
                    tunnel: w389 -> [w405]
                    tunnel: w388 -> [w404]
                    tunnel: w382 -> [w403]
                    tunnel: w387 -> [w402]
                    tunnel: w381 -> [w401]
                    tunnel: w386 -> [w400]
                    tunnel: w385 -> [w399]
                    tunnel: w380 -> [w398]
                    tunnel: w380 -> [w397]
                    tunnel: w384 -> [_]
                    tunnel: w383 -> [w444]
                    tunnel: w382 -> [w443]
                    tunnel: [w432] -> w377
                    tunnel: w379 -> [w435]
                    tunnel: [w431] -> w376
                    frame #0 {
                      n221 = case shown="假" w405 {
                        tunnel: w404 -> [w416 w430]
                        tunnel: w403 -> [w412 w429]
                        tunnel: w402 -> [w414 w428]
                        tunnel: w401 -> [_ w427]
                        tunnel: w400 -> [w411 _]
                        tunnel: w399 -> [w413 _]
                        tunnel: w398 -> [w410 _]
                        tunnel: w397 -> [w407 _]
                        frame False {
                          n222 = Not Equal?(x=w411, y=w414) -> (x != y?=w415:bool)
                          n223 = And(x=w415, y=w413) -> (x .and. y?=w409:bool)
                          n224 = Not(x=w407) -> (.not. x?=w406:bool)
                          n225 = And(x=w406, y=w409) -> (x .and. y?=w408:bool)
                          n226 = case shown="真" w408 {
                            tunnel: w416 -> [_ w423]
                            tunnel: w412 -> [_ w422]
                            tunnel: w411 -> [_ w421]
                            tunnel: w410 -> [_ w418]
                            frame False {
                            }
                            frame True {
                              n227 = Select(t=1, s=w418, f=0) -> (s? t:f=w417:i32)
                              n228 = call "ASI Set Control Value.vi"("bAuto"=w417, "lValue"=w421, "ControlType"=w422, "iCameraID"=w423) -> ()  [unwired: 7 in, 1 out]
                            }
                          }
                        }
                        frame True {
                          n229 = Select(t=1, s=w427, f=0) -> (s? t:f=w424:i32)
                          n230 = call "ASI Set Control Value.vi"("bAuto"=w424, "lValue"=w428, "ControlType"=w429, "iCameraID"=w430) -> ()  [unwired: 7 in, 1 out]
                        }
                      }
                    }
                    frame #1 {
                      n231 = call "ASI Get Control Value.vi"("ControlType"=w443, "iCameraID"=w444) -> ("plValue out"=w434:i32, "pbAuto out"=w441:i32)  [unwired: 7 in, 1 out]
                      n232 = local read "clusterOldCtrlVal"() -> (w442:cluster{"value":dbl, "auto":bool})
                      n233 = Greater?(x=w441, y=0) -> (0:w439:bool)
                      n234 = local read "cluster"() -> (w436:cluster{"name":string, "value":dbl, "auto":bool})
                      n235 = Select(t=TRUE, s=w439, f=FALSE) -> (s? t:f=w433:bool)
                      n236 = Bundle By Name(cluster=w442, "value"=w434, "auto"=w433) -> (w432:cluster{"value":dbl, "auto":bool})
                      n237 = Bundle By Name(cluster=w436, "name"=w435, "value"=w434, "auto"=w433) -> (w431:cluster{"name":string, "value":dbl, "auto":bool})
                    }
                  }
                }
                n238 = property on="OldCtrlVal[]" class="Arr (strict)"("Value"=w371) -> ()  [unwired: 2 in, 2 out]
                n239 = property on="newCtrlVal[]" class="Arr (strict)"("Value"=w370) -> ()  [unwired: 2 in, 2 out]
              }
            }
            n240 = local read "exit"() -> (w144:bool)
          }
          n241 = while {
            tunnel: w114 -> [w127]
            tunnel: cluster{dbl, "plValue out":dbl}[] [] -> [_]
            stop <- w134 stop-if-true
            n242 = Wait (ms)(milliseconds to wait=u32 1000 ("等待时间（毫秒）")) -> ()  [unwired: 1 out]
            n243 = property on="IsCoolerCam" class="DigNum (strict)"() -> ("Value"=w129:u32)  [unwired: 2 in, 2 out]
            n244 = call "ASI Get Control Value.vi"("ControlType"=8, "iCameraID"=w127) -> ("plValue out"=w132:i32)  [unwired: 7 in, 2 out]
            n245 = Equal?(x=w129, y=u8 1) -> (x = y?=w128:bool)
            n246 = Divide(x=w132, y=10) -> (x/y=w126:dbl)
            n247 = case shown="假" w128 {
              tunnel: w127 -> [_ w143]
              tunnel: w126 -> [w137 w141]
              tunnel: [w138 w139] -> w125
              frame False {
                n248 = Bundle(w137, 0) -> (w138:cluster{dbl, i32})  [unwired: 1 in]
              }
              frame True {
                n249 = call "ASI Get Control Value.vi"("ControlType"=15, "iCameraID"=w143) -> ("plValue out"=w140:i32)  [unwired: 7 in, 2 out]
                n250 = Bundle(w141, "plValue out"=w140) -> (w139:cluster{dbl, "plValue out":i32})  [unwired: 1 in]
              }
            }
            "temp and cool chart" <- w125
            n251 = local read "exit"() -> (w134:bool)
          }
        }
      }
    }
    frame #6 {
      n252 = local read "CameraID"() -> (w446:i32)
      n253 = local read "New Image"() -> (w445:T1)
      n254 = call "ASI Close Camera.vi"("iCameraID"=w446) -> ()  [unwired: 9 in, 2 out]
      n255 = call "IMAQ Dispose"("Image"=w445) -> ()  [unwired: 5 in, 1 out]
    }
  }
